vi "Methode3.vi"(8 "error in (no error)":errorcluster, 11 "Class ami in":refnum<class "Class ami.lvclass">) -> (0 "error out":errorcluster, 3 "Class ami out":refnum<class "Class ami.lvclass">)   [LabVIEW 2023, in "Class ami.lvclass"]
uses:
  Class ami.lvclass
  ID/ID.lvclass
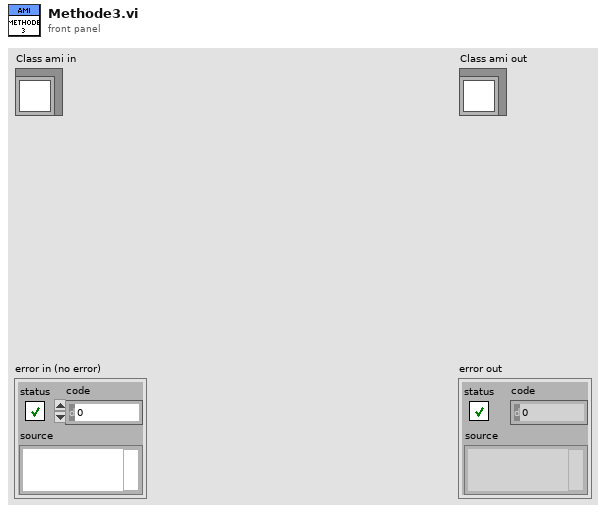
[diagram p1: front panel]
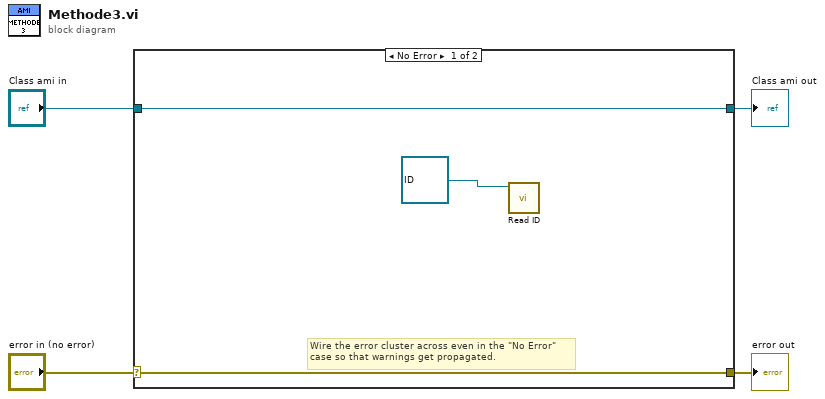
[diagram p0: block diagram]
diagram:
  n1 = case shown="No Error" "error in (no error)" {
    selector: "error in (no error)" -> [w7 w9]
    tunnel: [w7 w9] -> w3
    tunnel: [w6 w8] -> w1
    tunnel: "Class ami in" -> [w6 w8]
    frame No Error {
      # "Wire the error cluster across even in the \"No Error\"\ncase so that warnings get propagated."
      n2 = call-dynamic "Read ID.vi"("ID in"=refnum<class "ID.lvclass"> refnum ("ID.lvclass")) -> ()  [unwired: 8 in, 3 out]
    }
    frame Error {
    }
  }
  "error out" <- w3
  "Class ami out" <- w1
